vi "DIO 입출력 설정관리.vi"(11 "클러스터":cluster{"line grouping":i32, "lines":tag}={"line grouping"=1, "lines"=""} {"line grouping" items=["각 라인에 하나의 채널", "모든 라인에 하나의 채널"]}) -> (3 "출력 클러스터":cluster{"line grouping":i32, "lines":tag})   [LabVIEW 2022 SP3]
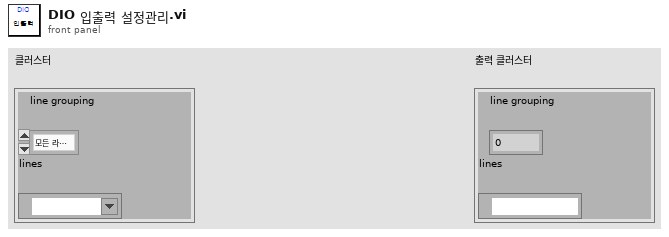
[diagram p1: front panel]
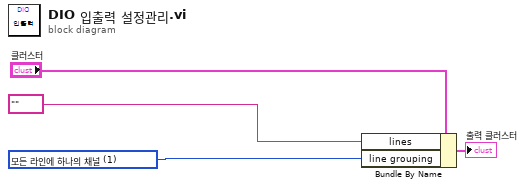
[diagram p0: block diagram]
diagram:
  w3 = 1 items=["각 라인에 하나의 채널", "모든 라인에 하나의 채널"] ("line grouping")
  n1 = Bundle By Name(cluster="클러스터", "lines"=tag "", "line grouping"=w3) -> (→"출력 클러스터":cluster{"line grouping":i32, "lines":tag})
